vi "create_control.vi"() -> ()   [LabVIEW 2014]
uses:
  <vilib>/National Instruments/iRobot Create/Advanced/UART/iRobot UART Port Type.ctl
  <vilib>/userdefined/High Color/IMAQdx.ctl
  <vilib>/vision/driver/NI_Vision_Acquisition_Software.lvlib
panel:
  in  "Session In":T1
  out "Image 2":T2(plugin-control)
  in  "stop":bool
  in  "stop 2":bool
  in  "Direction":dbl(slide) scale=-50.0..50.0
  in  "Speed":dbl(slide) scale=-50.0..50.0
  out "error out":errorcluster
  in  "Exit":bool
  out "Right Wheel":i32
  out "Left Wheel":i32
  in  "VISA resource name":T3
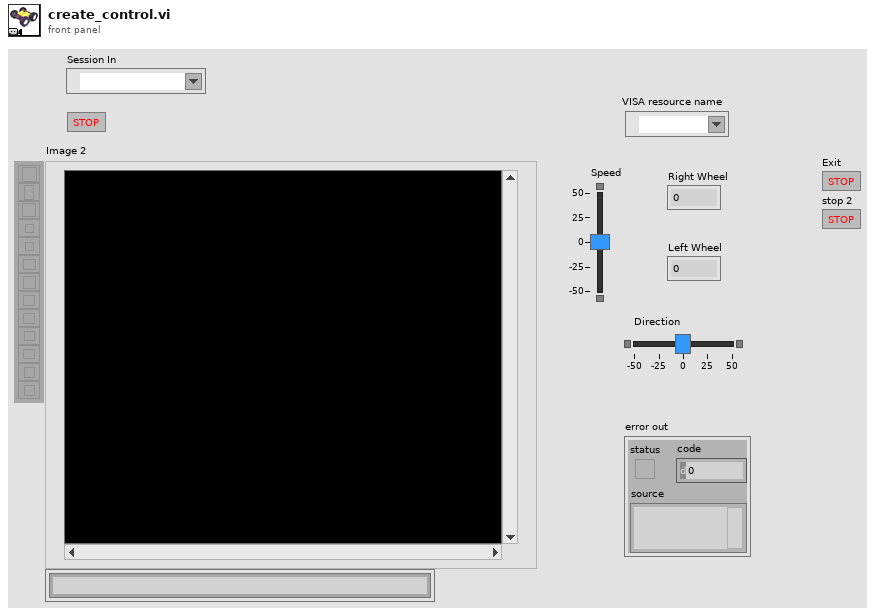
[diagram p1: front panel]
types:
  T1 = typedef "IMAQdx.ctl" = refnum<k21>
  T2 = typedef "IMAQ Image.ctl" = refnum<image>
  T3 = typedef "iRobot UART Port Type.ctl" = refnum<visa-resource-name>
  T4 = typedef "Image Type" = u32
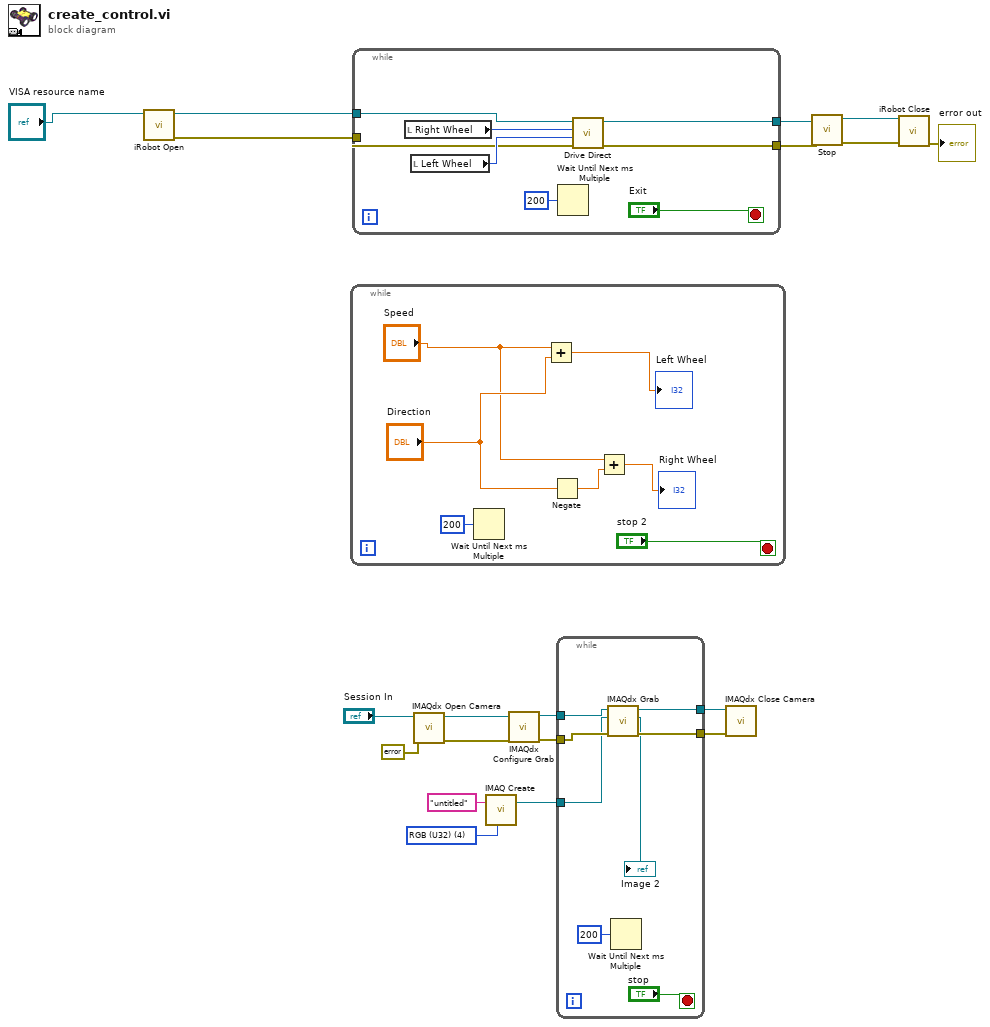
[diagram p0: block diagram]
diagram:
  w2 = T4 4 items=["Grayscale (U8)", "Grayscale (I16)", "Grayscale (SGL)", "Complex (CSG)", "RGB (U32)", "HSL (U32)", "RGB (U64)", "Grayscale (U16)"] ("Image Type")
  n1 = call <vilib>:"iRobot Open.vi"("UART port in"="VISA resource name") -> ("error out"=w17:errorcluster, "UART port out"=w18:T3)  [unwired: 9 in]
  n2 = while {
    stop <- "stop 2" stop-if-true
    n3 = Wait Until Next ms Multiple(millisecond multiple=u32 200) -> ()  [unwired: 1 out]
    n4 = Add(x="Speed", y="Direction") -> (x+y=→"Left Wheel":dbl)
    n5 = Negate(x="Direction") -> (-x=w23:dbl)
    n6 = Add(x="Speed", y=w23) -> (x+y=→"Right Wheel":dbl)
  }
  n7 = while {
    tunnel: w18 -> [w32]
    tunnel: w17 -> [w31]
    tunnel: [w30] -> w15
    tunnel: [w29] -> w16
    stop <- "Exit" stop-if-true
    n8 = local read "Right Wheel"() -> (w34:i32)
    n9 = local read "Left Wheel"() -> (w33:i32)
    n10 = Wait Until Next ms Multiple(millisecond multiple=u32 200) -> ()  [unwired: 1 out]
    n11 = call <vilib>:"Drive Direct.vi"("error in"=w31, "Left Wheel Velocity (mm/s)"=w33, "Right Wheel Velocity (mm/s)"=w34, "UART port in"=w32) -> ("error out"=w30:errorcluster, "UART port out"=w29:T3)  [unwired: 6 in]
  }
  n12 = call <vilib>:"IMAQdx Open Camera.vi"("error in"=errorcluster {"status"=FALSE, "code"=0, "source"=""}, "Session In"="Session In") -> ("error out"=w8:errorcluster, "Session Out"=w9:T1)  [unwired: 8 in]
  n13 = call "IMAQ Create"("Image Name"="untitled", "Image Type"=w2) -> ("New Image"=w1:T2)  [unwired: 3 in, 1 out]
  n14 = call <vilib>:"IMAQdx Configure Grab.vi"("error in"=w8, "Session In"=w9) -> ("error out"=w6:errorcluster, "Session Out"=w7:T1)  [unwired: 8 in]
  n15 = while {
    tunnel: w7 -> [w42]
    tunnel: w6 -> [w41]
    tunnel: [w40] -> w5
    tunnel: [w39] -> w4
    tunnel: w1 -> [w38]
    stop <- "stop" stop-if-true
    n16 = call <vilib>:"IMAQdx Grab.vi"("error in"=w41, "Image In"=w38, "Session In"=w42) -> ("error out"=w39:errorcluster, "Image Out"=→"Image 2":T2, "Session Out"=w40:T1)  [unwired: 5 in, 1 out]
    n17 = Wait Until Next ms Multiple(millisecond multiple=u32 200) -> ()  [unwired: 1 out]
  }
  n18 = call <vilib>:"IMAQdx Close Camera.vi"("error in"=w4, "Session In"=w5) -> ()  [unwired: 9 in, 1 out]
  n19 = call <vilib>:"Stop.vi"("error in"=w15, "UART port in"=w16) -> ("error out"=w13:errorcluster, "UART port out"=w14:T3)  [unwired: 8 in]
  n20 = call <vilib>:"iRobot Close.vi"("error in"=w13, "UART port in"=w14) -> ("error out"=→"error out":errorcluster)  [unwired: 9 in]
